vi "Globals.vi"() -> ()   [LabVIEW 2018]
panel:
  in  "AutoOverride":bool
  in  "ManualOverride":bool
  in  "AutoClimb":bool
  in  "CargoShipAlign":bool
  in  "ClimbStage":T1(ring)
  out "DisplaceOffsets":dbl[](array[numeric])
  out "Velocity":dbl
  in  "ZeroHatch":bool
  in  "ReleaseCargo":bool
  in  "IRDistance":dbl
  out "ErrorMessage":string
  out "LiftLevel":enum16{"Low", "Mid", "High"}(ring)
  in  "ArmOut":bool
  in  "ReleaseHatch":bool
  in  "ZeroGyro":bool
  in  "VisionAlign":bool
  in  "DriveMode":enum16{"Swerve", "Ackerman"}(ring)
  in  "Gyro":dbl
  in  "ZAxis":dbl
  in  "YAxis":dbl
  in  "XAxis":dbl
  # "Code:"
  # "Pilot:"
  # "Copilot:"
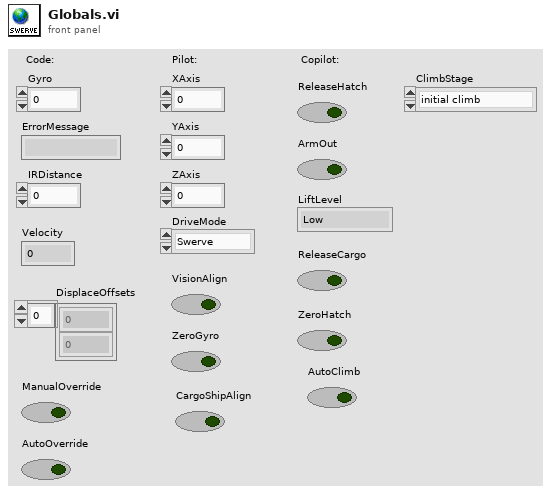
[diagram p1: front panel]
types:
  T1 = enum16{"initial climb", "elevated drive", "retract 1", "on platform drive", "retract 2", "finish"}
diagram:
